vi "WLAN - Test - UTIL - Power Level Settings.vi"(0 "Sweep Settings":T1) -> (4 "# of Power Levels":i32, 6 "Power Level Settings.Start Power Level(dBm)":dbl, 10 "Power Level Settings.Step Size":dbl)   [LabVIEW 2011]
uses:
  TV/RW/Includes/WLAN - TV - RW - INC - Rx_PER_Sweep_Settings.ctl
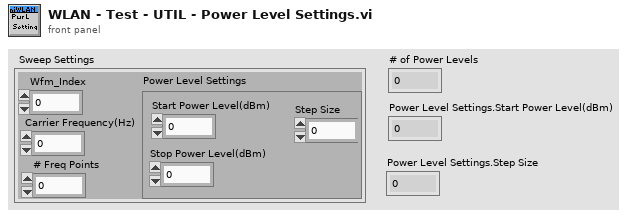
[diagram p1: front panel]
types:
  T1 = typedef "WLAN - TV - RW - INC - Rx_PER_Sweep_Settings.ctl" = cluster{"Wfm_Index":i32, "Power Level Settings":cluster{"Stop Power Level(dBm)":dbl, "Start Power Level(dBm)":dbl, "Step Size":dbl}, "Carrier Frequency(Hz)":dbl, "# Freq Points":i32}
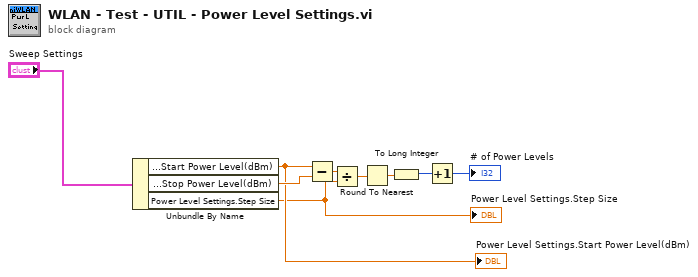
[diagram p0: block diagram]
diagram:
  n1 = Unbundle By Name("Sweep Settings") -> ("Power Level Settings.Start Power Level(dBm)"=w5:dbl, "Power Level Settings.Stop Power Level(dBm)"=w9:dbl, "Power Level Settings.Step Size"=w1:dbl)
  "Power Level Settings.Step Size" <- w1
  "Power Level Settings.Start Power Level(dBm)" <- w5
  n2 = Subtract(x=w5, y=w9) -> (x-y=w8:dbl)
  n3 = Divide(x=w8, y=w1) -> (x/y=w7:dbl)
  n4 = Round To Nearest(number=w7) -> (nearest integer value=w6:dbl)
  n5 = To Long Integer(number=w6) -> (32bit integer=w3:i32)
  n6 = Increment(x=w3) -> (x+1=→"# of Power Levels":i32)
